vi "From JSON String.vi"(8 "error in":errorcluster, 10 "JSON String":string, 11 "Configuration Base in":refnum<class "Configuration Base.lvclass">) -> (0 "error out":errorcluster, 3 "Configuration Base out":refnum<class "Configuration Base.lvclass">)   [LabVIEW 2023, in "HAL.lvlib" / "Configuration Base.lvlib" / "Configuration Base.lvclass"]
uses:
  Configuration Base.lvclass
  Configuration Base.lvclass/Configuration Base.ctl
  <vilib>/Utility/error.llb/Error Cluster From Error Code.vi
  <vilib>/ErrorRing/Error Ring.xnode
  <vilib>/JDP Science/JSONtext/JSONtext.lvlib
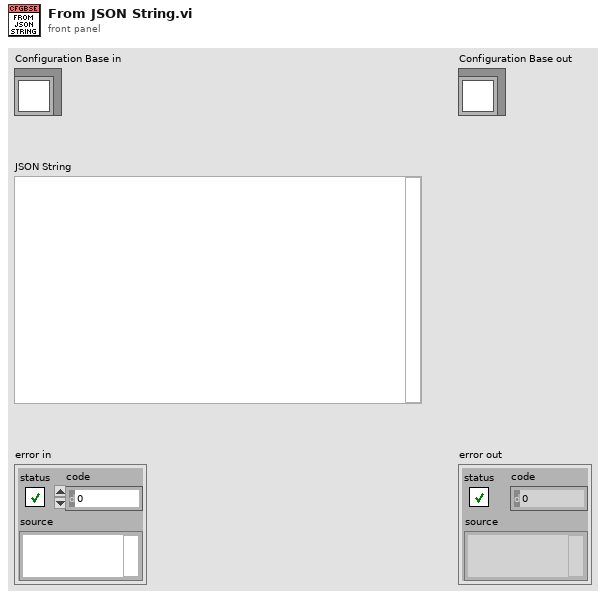
[diagram p1: front panel]
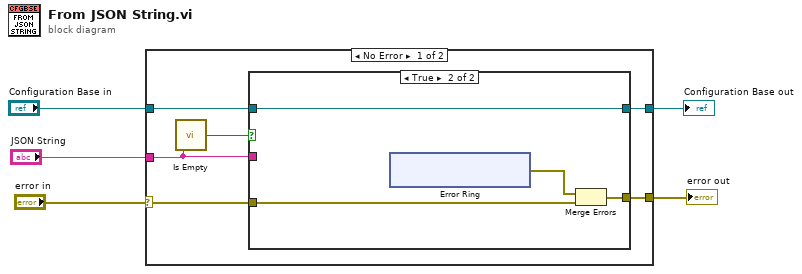
[diagram p0: block diagram]
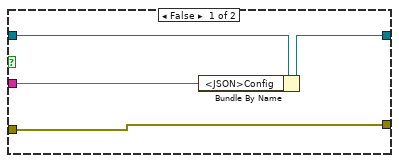
[diagram p2: hidden frame]
diagram:
  n1 = case shown="No Error" "error in" {
    selector: "error in" -> [w7 w26]
    tunnel: [w10 w26] -> w4
    tunnel: [w9 w25] -> w3
    tunnel: "Configuration Base in" -> [w11 w25]
    tunnel: "JSON String" -> [w6 _]
    frame No Error {
      n2 = call <vilib>:"Is Empty.vi"("JSON"=w6) -> ("Empty"=w8:bool)  [unwired: 4 in]
      n3 = case shown="True" w8 {
        tunnel: w11 -> [w15 w16]
        tunnel: [w13 w16] -> w9
        tunnel: w7 -> [w14 w17]
        tunnel: [w14 w19] -> w10
        tunnel: w6 -> [w12 _]
        frame False {
          n4 = Bundle By Name(cluster=w15, "<JSON>Config"=w12) -> (w13:refnum<class "Configuration Base.lvclass">)
        }
        frame True {
          n5 = xnode "Error Ring"() -> ("error out"=w18:errorcluster)
          n6 = Merge Errors(w18, w17) -> (w19:errorcluster)
        }
      }
    }
    frame Error {
    }
  }
  "error out" <- w4
  "Configuration Base out" <- w3
